vi "RegisterCurrentServer.vi"(2 "ROS in":T1={"topic port"=0, "Node"="", "topic"="", "type"="", "node port"=0, "error "={"status"=FALSE, "code"=0, "source"=""}, "Direction"=enum."Node", "APIs"=[], "Update (ms)"=1, "write queue"=1}, 3 "This VI":refnum<vi>) -> (0 "ROS out":T1={"topic port"=0, "Node"="", "topic"="", "type"="", "node port"=0, "error "={"status"=FALSE, "code"=0, "source"=""}, "Direction"=enum."Node", "APIs"=[], "Update (ms)"=1, "write queue"=1})   [LabVIEW 2010]
uses:
  _ROSDefinition.vi
  SubVIs/_ROSDirection.ctl
  SubVIs/_ROSControl.ctl
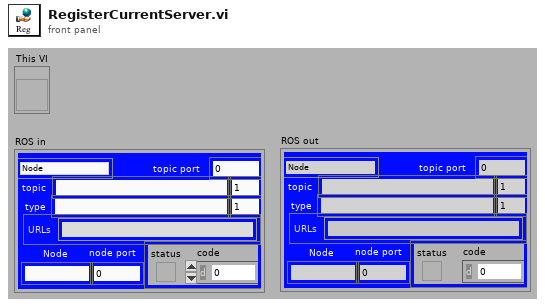
[diagram p1: front panel]
types:
  T1 = typedef "_ROSControl.ctl" = cluster{"topic port":u16, "Node":string, "topic":string, "type":string, "node port":u32, "error ":errorcluster, "Direction":T2, "APIs":string[], "Update (ms)":u16, "write queue":u16}
  T2 = typedef "_ROSDirection.ctl" = enum16{"Node", "Publisher", "Subscriber", "Service Client"}
  T3 = enum16{"Add Server", "Clear Server", "Clear All", "Get Info"}
  T4 = cluster{"vi name":string, "This VI":refnum<vi>, "queue out":refnum<queue>, "ROS in":T1, "notifier out":refnum<notifier>}
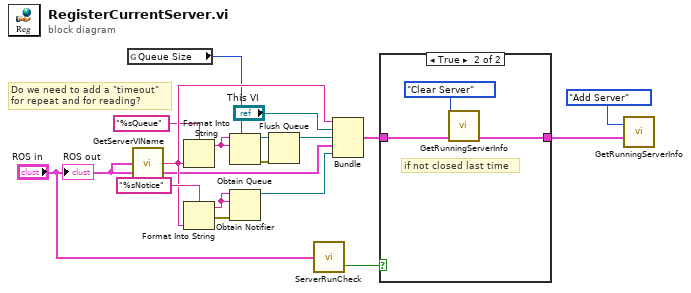
[diagram p0: block diagram]
diagram:
  # "Do we need to add a \"timeout\"\nfor repeat and for reading?"
  n1 = global read "_ROSDefinition.vi" "Queue Size"() -> (w1:i32)
  n2 = call "GetServerVIName.vi"("ROS"="ROS in") -> ("vi name"=w12:string)
  n3 = Format Into String(format string="%sQueue" ("name (unnamed)"), w12) -> (resulting string=w10:string)  [unwired: 2 in, 1 out]
  n4 = Format Into String(format string="%sNotice" ("name (unnamed)"), w12) -> (resulting string=w14:string, error out=w11:errorcluster)  [unwired: 2 in]
  n5 = Obtain Queue(max queue size (-1, unlimited)=w1, name (unnamed)=w10, element data type=w10) -> (queue out=w4:refnum<queue>, error out=w2:errorcluster)  [unwired: 2 in, 1 out]
  n6 = Obtain Notifier(name (unnamed)=w14, notification data type=w14, error in (no error)=w11) -> (notifier out=w15:refnum<notifier>)  [unwired: 1 in, 2 out]
  n7 = Flush Queue(queue=w4, error in (no error)=w2) -> (queue out=w3:refnum<queue>)  [unwired: 2 out]
  n8 = call "ServerRunCheck.vi"("ROS in"="ROS in") -> ("Running?"=w8:bool)  [unwired: 1 out]
  n9 = Bundle("vi name"=w12, "This VI"="This VI", "queue out"=w3, "ROS in"="ROS in", "notifier out"=w15) -> (w16:T4)  [unwired: 1 in]
  n10 = case shown="True" w8 {
    tunnel: w16 -> [w18 w19]
    tunnel: [w18 w19] -> w6
    frame False {
    }
    frame True {
      # "if not closed last time"
      n11 = call "GetRunningServerInfo.vi"("New Server"=w19, "Task"=T3."Clear Server") -> ()  [unwired: 3 out]
    }
  }
  n12 = call "GetRunningServerInfo.vi"("New Server"=w6, "Task"=T3."Add Server") -> ()  [unwired: 3 out]
  "ROS out" <- "ROS in"
